vi "Read Profiles(for Advanced Mode).vi"(0 "Device ID (0)":i32, 9 "Data Size (0: Auto Size)":u32, 11 "error in (no error)":errorcluster) -> (3 "Profile Info":T4, 4 "Device ID out":i32, 6 "Profile Data":u32[](array[numeric]), 14 "Measure Data":T1[](array[typedef]) {"Judge Result" items=["HI", "GO", "LO", "ALARM"]; "Data Info" items=["VALID", "ALARM", "WAIT"]}, 15 "error out":errorcluster)   [LabVIEW 8.6, in "Keyence LJ-V7000.lvlib"]
doc: "This function gets profile data.\nProfile data is stored in 0.01 μm units.\n\n<B>Note</B>:\n For the details on the data stored in the profile data (storage order and size), see <B>10.3</B> in a manual of measuring instrument drivers."
uses:
  Keyence LJ-V7000.lvlib
  constant/Driver VI No.ctl
  Clusters/Profile Info.ctl
  constant/Judge Result.ctl
  constant/Measure Data Info.ctl
  Clusters/Measure Data.ctl
panel:
  # "(c) 2012 KEYENCE CORPORATION.  ALL RIGHTS RESERVED."
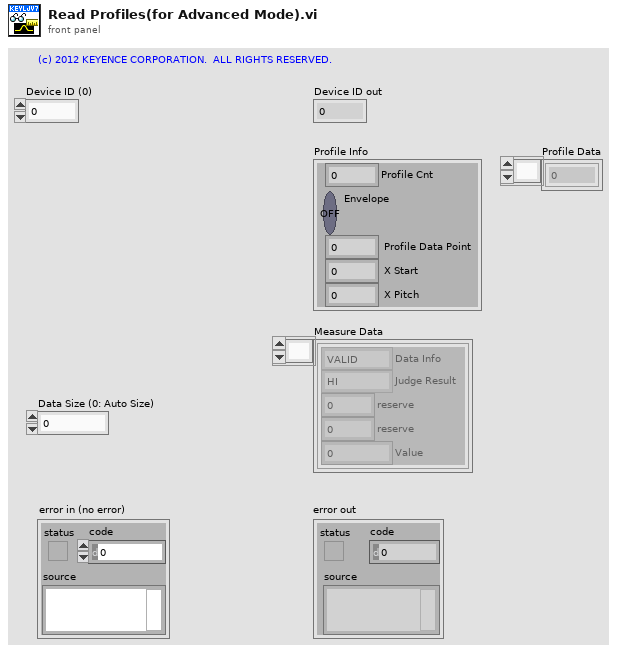
[diagram p1: front panel]
types:
  T1 = typedef "Keyence LJ-V7000.lvlib/Measure Data.ctl" = cluster{"Data Info":T2, "Judge Result":T3, "reserve":u8, "reserve":u8, "Value":sgl}
  T2 = typedef "Keyence LJ-V7000.lvlib/Measure Data Info.ctl" = u8
  T3 = typedef "Keyence LJ-V7000.lvlib/Judge Result.ctl" = u8
  T4 = typedef "Keyence LJ-V7000.lvlib/Profile Info.ctl" = cluster{"Profile Cnt":u8, "Envelope":bool, " Profile Data Point":u16, " X Start":i32, " X Pitch":i32}
  T5 = typedef "Keyence LJ-V7000.lvlib/Driver VI No.ctl" = enum16{"Initialize", "Close", "Reboot Controller", "Return to Factory State", "Get System Error", "Clear System Error", "Trigger", "Start Batch Measurements", "Stop Batch Measurements", "Auto Zero", "Timing", "Reset", "Clear Memory", "Set Setting", "Get Setting", "Initialize Setting", "Reflect Setting", "Update Write Settings Area", "Check Status of Saving to Save Area", "Set Time", "Get Time", "Change Program", "Read Active Program Number", "Read Measurement Data", "Read Profiles(for High-Speed Mode)", "Read Batch Profiles(for High-Speed Mode)", "Read Profiles(for Advanced Mode)", "Read Batch Profiles(for Advanced Mode)", "Start Storage", "Stop Storage", "Read Storage Status", "Read Data Storage Data", "Read Profile Storage Data", "Read Batch Profile Storage Data", "Start High-Speed Data Communication", "Stop High-Speed Data Communication", "Read Profiles(for High-Speed Communication)"}
  T6 = cluster{"Profile Cnt":u8, u8, "reserve":u8, "reserve":u8, " Profile Data Point":u16, "reserve":u8, "reserve":u8, " X Start":i32, " XPitch":i32}
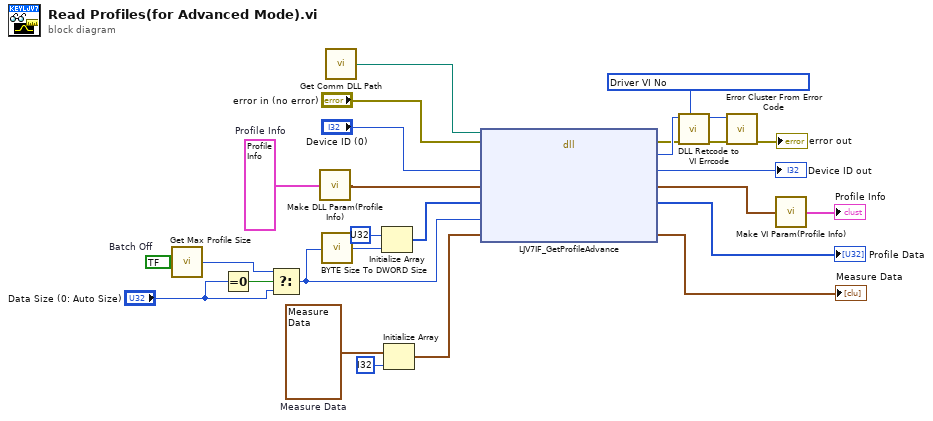
[diagram p0: block diagram]
diagram:
  w6 = bool ?  # Batch Off
  w18 = T1 ?  # Measure Data
  w21 = T4 ?  # Profile Info
  n1 = call "Get Max Profile Size.vi"("Batch On-Off"=w6) -> ("Profile Size"=w3:u32)  [unwired: 4 in]
  n2 = Equal To 0?(x="Data Size (0: Auto Size)") -> (x = 0?=w7:bool)
  n3 = Select(t=w3, s=w7, f="Data Size (0: Auto Size)") -> (s? t:f=w1:u32)
  n4 = call "Make DLL Param(Profile Info).vi"("Profile Info"=w21) -> ("DLL Parameter"=w22:T6)
  n5 = call "BYTE Size To DWORD Size.vi"("BYTE Size"=w1) -> ("DWORD Size"=w2:u32)
  n6 = call "Get Comm DLL Path.vi"() -> ("Comm DLL Path"=w25:path)  [unwired: 1 in]
  n7 = Initialize Array(u32 ?, w2) -> (w5:u32[])
  n8 = Initialize Array(w18, i32 ? ("次元サイズ")) -> (w16:T1[])
  n9 = dll-call lib="C:/Program Files/National Instruments/LabVIEW 2011/instr.lib/Keyence LJ-V7000/LJV7_IF.*" fn="LJV7IF_GetProfileAdvance"(path in=w25, error in="error in (no error)", "lDeviceId"="Device ID (0)", "pProfileInfo"=w22, "pdwProfileData"=w5, "dwDataSize"=w1, "pMeasureData"=w16) -> (error out=w11:errorcluster, "lRetCode"=w12:i32, "lDeviceId"=→"Device ID out":i32, "pProfileInfo"=w20:T6, "pdwProfileData"=→"Profile Data":u32[], "pMeasureData"=→"Measure Data":T1[])  [unwired: 2 in, 1 out]
  n10 = call "DLL Retcode to VI Errcode.vi"("Driver VI No"=T5 ?, "error in (no error)"=w11, "DLL Return Code"=w12) -> ("error out"=w14:errorcluster, "VI Error Code"=w13:i32)  [unwired: 7 in]
  n11 = call <vilib>:"Error Cluster From Error Code.vi"("error in (no error)"=w14, "error code (0)"=w13) -> ("error out"=→"error out":errorcluster)  [unwired: 7 in]
  n12 = call "Make VI Param(Profile Info).vi"("pProfileInfo"=w20) -> ("Profile Info"=→"Profile Info":T4)
